vi "Subtract Float SCTL 40 MHz Latency 0 Pipeline 0.vi"(1 "y":sgl, 2 "x":sgl) -> (0 "x-y":sgl)   [LabVIEW 2014]
uses:
  <vilib>/rvi/IPIntegrationNode/IPINode_Typedef/niFpgaIPINodeSupportedFamilies.ctl
  <vilib>/rvi/IPIntegrationNode/IPINode_Utilities/niFpgaIPINodeSimCore.vi
  <vilib>/rvi/XilinxIP/XIPIN_XNode/niFpgaXIPIN.xnode
  Coregen SPARTAN6/Subtract SCTL L0/Subtract_SCTL_L0_C3ADE5BE76064AA39E7EE6565DE88692.dll
  <vilib>/rvi/IPIntegrationNode/IPINode_Xnode/niFpgaIPINode.xnode
  Coregen Zynq/Subtract SCTL L0/xsim.dir/Subtract_SCTL_L0_FF5539BE3A844865B6741F57DA4DC489/xsimk_FF5539BE3A844865B6741F57DA4DC489.dll
  Coregen KINTEX7/Subtract SCTL L0/xsim.dir/Subtract_SCTL_L0_614AA3EEFEF54D979388EDD38958139F/xsimk_614AA3EEFEF54D979388EDD38958139F.dll
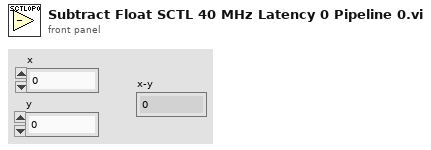
[diagram p1: front panel]
types:
  T1 = typedef "niFpgaIPINodeSupportedFamilies.ctl" = cluster{"unlimited?":bool, "supported targets":string[]}
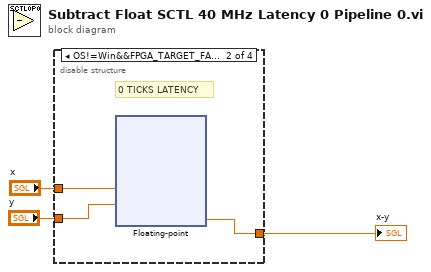
[diagram p0: block diagram]
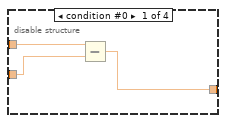
[diagram p2: hidden frame]
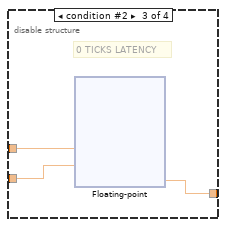
[diagram p3: hidden frame]
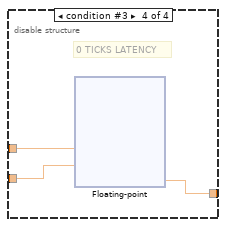
[diagram p4: hidden frame]
diagram:
  n1 = disable-structure shown="OS!=Win&&FPGA_TARGET_FAMILY==SPARTAN6" {
    disable-tunnel: "x" -> [w6 w9 w66 w129]
    disable-tunnel: [w4 w7 w64 w127] -> w1
    disable-tunnel: "y" -> [w5 w8 w65 w128]
    frame condition #0 {
      n2 = Subtract(x=w6, y=w5) -> (x-y=w4:sgl)
    }
    frame condition #1 (active) {
      # "0 TICKS LATENCY"
      n3 = xnode ("Floating-point")("a"=w9, "b"=w8) -> ("result"=w7:sgl)
    }
    frame condition #2 {
      # "0 TICKS LATENCY"
      n4 = xnode ("Floating-point")("s_axis_a_tdata"=w66, "s_axis_b_tdata"=w65) -> ("m_axis_result_tdata"=w64:sgl)  [unwired: 2 in, 1 out]
    }
    frame condition #3 {
      # "0 TICKS LATENCY"
      n5 = xnode ("Floating-point")("s_axis_a_tdata"=w129, "s_axis_b_tdata"=w128) -> ("m_axis_result_tdata"=w127:sgl)  [unwired: 2 in, 1 out]
    }
  }
  "x-y" <- w1
